vi "Actor Core.vi"(8 "error in":errorcluster, 11 "WS Test Client in":refnum<class "WS Client.lvclass">) -> (0 "error out":errorcluster, 3 "Actor out":refnum<class "Actor.lvclass">)   [LabVIEW 2021, in "Echo Broadcast Without Server Manager.lvlib" / "WS Client.lvclass"]
doc: "(<B>Filename</B>: Actor Framework.lvlib:Actor.lvclass:Actor Core.vi)\n\nReceives messages to the actor, reacts to them, and initiates any error handling that may shut the actor down.\n\nDescendant classes may override this VI to append parallel tasks for the actor to complete while it handles messages. Overrides use the Call Parent Method node."
uses:
  WS Client.lvclass
  <vilib>/ActorFramework/Actor/Actor.lvclass
  <vilib>/ActorFramework/Message Enqueuer/Message Enqueuer.lvclass
  WS Client.lvclass/WS Client.ctl
  WebSocket Actor/WebSocket Connection Messages/Send to Peer Msg/Send to Peer Msg.lvclass
  <userlib>/_OpenG.lib/error/error.llb/openg_error.lvlib
panel:
  in  "Send":bool
  in  "Data To Send":string
  out "Echoed Data":string
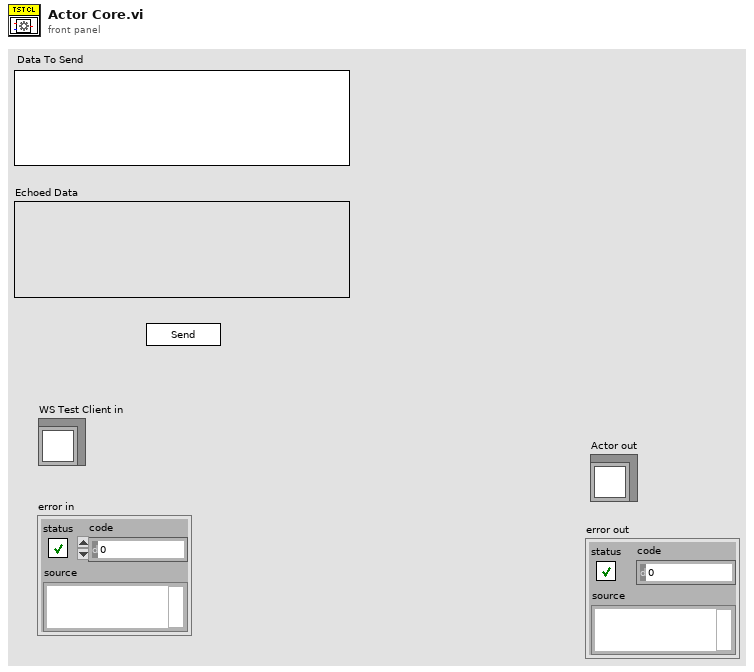
[diagram p1: front panel]
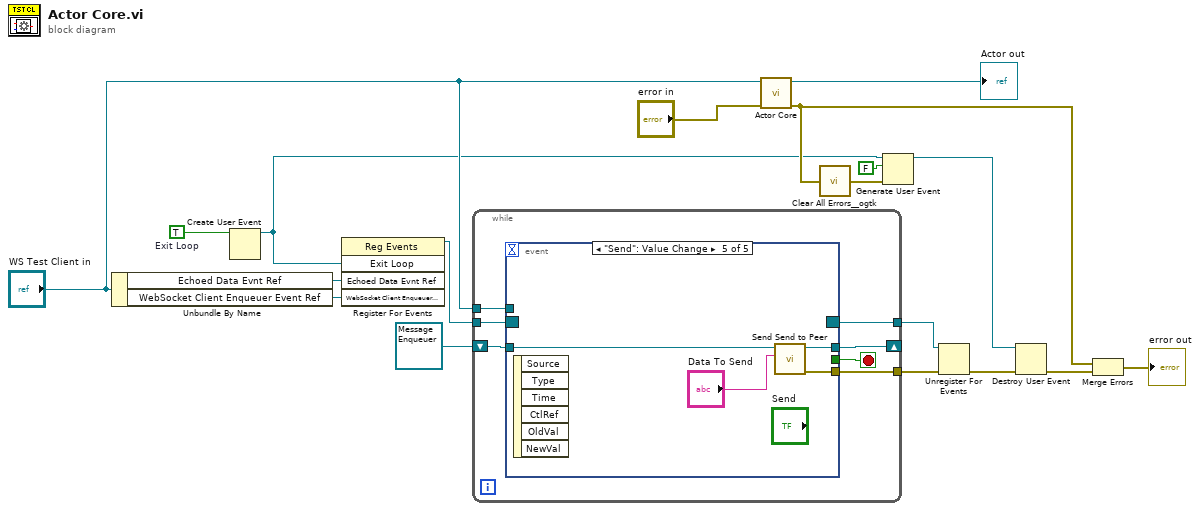
[diagram p0: block diagram]
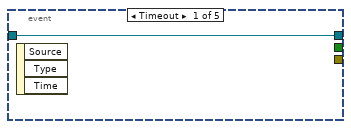
[diagram p2: hidden frame]
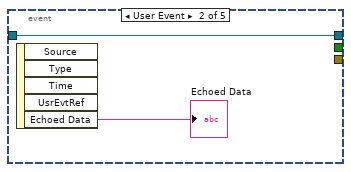
[diagram p3: hidden frame]
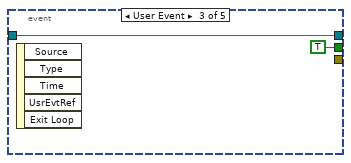
[diagram p4: hidden frame]
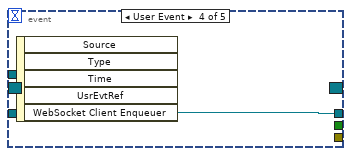
[diagram p5: hidden frame]
diagram:
  w8 = TRUE  # Exit Loop
  n1 = Unbundle By Name("WS Test Client in") -> ("Echoed Data Evnt Ref"=w16:refnum<user-event>, "WebSocket Client Enqueuer Event Ref"=w14:refnum<user-event>)
  n2 = Create User Event(user event datatype=w8) -> (user event=w1:refnum<user-event>)  [unwired: 1 in, 1 out]
  n3 = register-events(w1, w16, w14) -> (reference out=w15:refnum<event-registration>)  [unwired: 2 in, 1 out]
  n4 = while {
    tunnel: w15 -> [w25]
    shift-right: [w23] -> _
    shift-left: refnum<class "Message Enqueuer.lvclass"> refnum ("WebSocket Client Enqueuer") -> [w22]
    tunnel: [w21] -> w12
    tunnel: "WS Test Client in" -> [w20]
    tunnel: [w19] -> w9
    stop <- w24 stop-if-true
    n5 = event shown="[4] \"Send\": Value Change" {
      selector: w25 -> [_ _ _ _ _]
      dyn-events: [_ _ _ _ _] -> w21
      timeout: _ -> [_ _ _ _ _]
      tunnel: [_ _ TRUE ("Exit") _ _] -> w24
      tunnel: [w26 w27 w30 w31 w33] -> w23
      tunnel: w22 -> [w26 w27 w30 _ w34]
      tunnel: w20 -> [_ _ _ _ _]
      tunnel: [_ _ _ _ w32] -> w19
      event Timeout {
        n6 = event-data() -> ()  [unwired: 1 in, 3 out]
      }
      event User Event {
        n7 = event-data() -> ("Echoed Data"=→"Echoed Data":string)  [unwired: 1 in, 4 out]
      }
      event User Event {
        n8 = event-data() -> ()  [unwired: 1 in, 5 out]
      }
      event User Event {
        n9 = event-data() -> ("WebSocket Client Enqueuer"=w31:refnum<class "Message Enqueuer.lvclass">)  [unwired: 1 in, 4 out]
      }
      event "Send": Value Change {
        n10 = event-data() -> ()  [unwired: 1 in, 6 out]
        n11 = call "Send Send to Peer.vi"("Data"="Data To Send", "Message Enqueuer in"=w34) -> ("error out"=w32:errorcluster, "Message Enqueuer out"=w33:refnum<class "Message Enqueuer.lvclass">)  [unwired: 8 in]
      }
    }
  }
  n12 = call-parent "Actor Core.vi"("error in"="error in", "Actor in"="WS Test Client in") -> ("error out"=w4:errorcluster, "Actor out"=→"Actor out":refnum<class "Actor.lvclass">)  [unwired: 8 in]
  n13 = call <userlib>:"Clear All Errors__ogtk.vi"("Error In"=w4) -> ("Error Out"=w7:errorcluster)  [unwired: 3 in]
  n14 = Generate User Event(user event=w1, event data cluster=FALSE ("event data"), error in=w7) -> (user event out=w5:refnum<user-event>)  [unwired: 1 in, 1 out]
  n15 = Unregister For Events(event registration refnum=w12, error in=w9) -> (error out=w3:errorcluster)
  n16 = Destroy User Event(user event=w5, error in=w3) -> (error out=w2:errorcluster)
  n17 = Merge Errors(w4, w2) -> (→"error out":errorcluster)
